vi "FTW-Test-JSON-Stress.vi"() -> (0 "Test Result":errorcluster)   [LabVIEW 2015]
panel:
  out "Serialized JSON":string[](array[string])
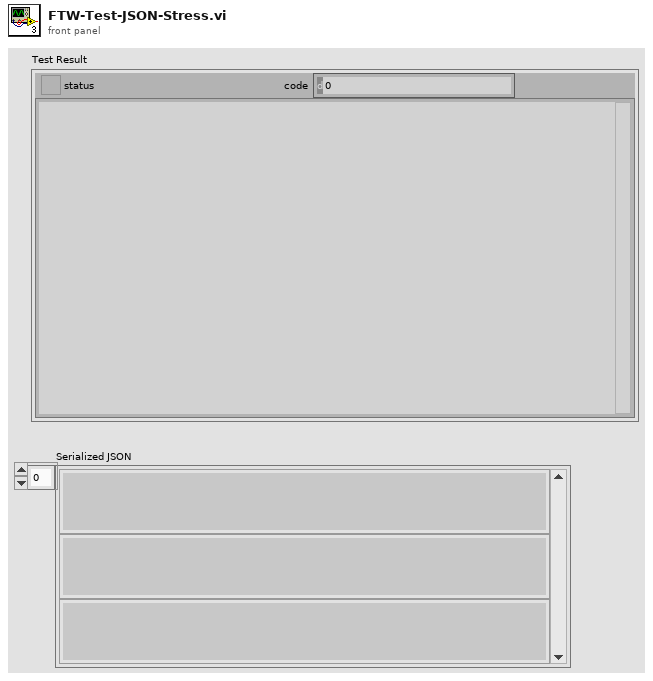
[diagram p1: front panel]
types:
  T1 = typedef "FTW-Type-JSON.ctl" = refnum<data-value>
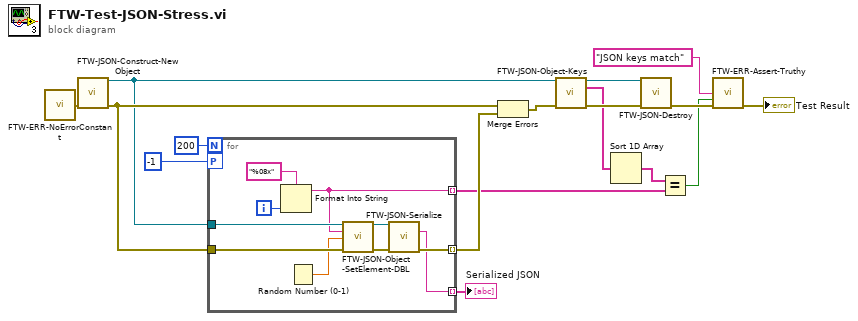
[diagram p0: block diagram]
diagram:
  n1 = call "FTW-ERR-NoErrorConstant.vi"() -> ("no error"=w7:errorcluster)
  n2 = call "FTW-JSON-Construct-NewObject.vi"("error in"=w7) -> ("JSON"=w14:refnum<class "FTW-Container.lvclass">, "error out"=w15:errorcluster)  [unwired: 13 in]
  n3 = for {
    N: 200 -> [_]
    tunnel: [w23] -> w4 mode=indexing
    workers-P: -1 -> [_]
    tunnel: w15 -> [w26]
    tunnel: [w25] -> w16 mode=indexing
    tunnel: w14 -> [w27]
    tunnel: [w18] -> w12 mode=indexing
    i -> [w19]
    n4 = Format Into String(format string="%08x", w19) -> (resulting string=w18:string)  [unwired: 2 in, 1 out]
    n5 = Random Number (0-1)() -> (number: 0 to 1=w24:dbl)
    n6 = call "FTW-JSON-Object-SetElement-DBL.vi"("JSON"=w27, "Key"=w18, "Value"=w24, "error in"=w26) -> ("JSON out"=w22:refnum<class "FTW-Container.lvclass">, "error out"=w21:errorcluster)  [unwired: 10 in]
    n7 = call "FTW-JSON-Serialize.vi"("JSON"=w22, "error in"=w21) -> ("JSON String (UTF-8)"=w23:string, "error out"=w25:errorcluster)  [unwired: 11 in, 1 out]
  }
  "Serialized JSON" <- w4
  n8 = Merge Errors(w15, w16) -> (w13:errorcluster)
  n9 = call "FTW-JSON-Object-Keys.vi"("JSON"=w14, "error in"=w13) -> ("JSON out"=w11:T1, "Keys"=w6:string[], "error out"=w10:errorcluster)  [unwired: 11 in]
  n10 = Sort 1D Array(array=w6) -> (sorted array=w5:string[])
  n11 = call "FTW-JSON-Destroy.vi"("JSON"=w11, "error in"=w10) -> ("error out"=w9:errorcluster)  [unwired: 13 in]
  n12 = Equal?(x=w5, y=w12) -> (x = y?=w2:bool)
  n13 = call "FTW-ERR-Assert-Truthy.vi"("Assertion"="JSON keys match", "Assertion holds true?"=w2, "error in"=w9) -> ("error out"=→"Test Result":errorcluster)  [unwired: 12 in]
